vi "Test - Parse Cluster.vi"() -> ()   [LabVIEW 2020, in "JSON Schema Generator.lvlib"]
uses:
  JSON Schema Generator.lvlib
  <vilib>/addons/_JKI Toolkits/Caraya/classes/Test/Test.lvclass
  <vilib>/addons/_JKI Toolkits/Caraya/classes/Assert/Assert.lvclass
  <vilib>/JDP Science/JSONtext/JSONtext.lvlib
  <vilib>/addons/_JKI Toolkits/Caraya/classes/Assert/Assert Equal Value_Variant.vi
  <vilib>/addons/_JKI Toolkits/Caraya/classes/Assert/Assert Not Error.vi
panel:
  out "Typedef Name":string
  out "JSON Object Name":string
  in  "A Cluster":T1
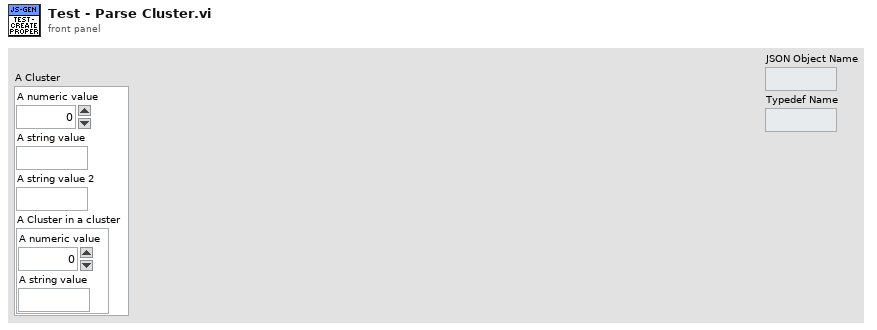
[diagram p1: front panel]
types:
  T1 = cluster{"A numeric value":i32, "A string value":string, "A string value 2":string, "A Cluster in a cluster":cluster{"A numeric value":i32, "A string value":string}}
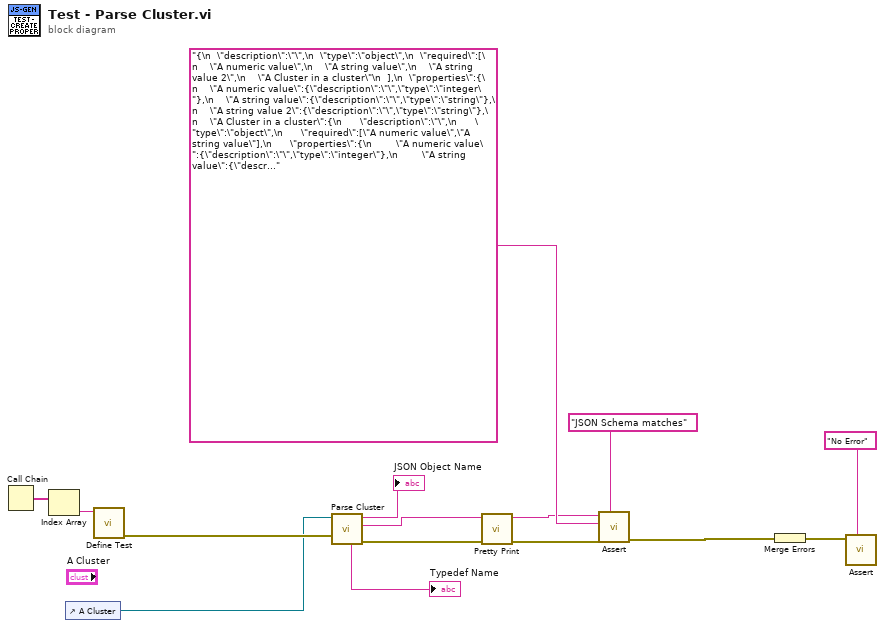
[diagram p0: block diagram]
diagram:
  n1 = Call Chain() -> (call chain=w15:string[])
  n2 = Index Array(array=w15) -> (element=w14:string)  [unwired: 1 in]
  n3 = control-ref of="A Cluster"() -> (w3:refnum<vi>)
  n4 = call <vilib>:"Define Test.vi"("Label (VI Title)"=w14) -> ("error out"=w9:errorcluster)  [unwired: 9 in, 1 out]
  n5 = call "Parse Cluster.vi"("error in"=w9, "Cluster Refnum In"=w3) -> ("error out"=w5:errorcluster, "JSON ObjectSchema out"=w8:string, "JSON Object Name"=→"JSON Object Name":string, "Typedef Name"=→"Typedef Name":string)  [unwired: 5 in, 1 out]
  n6 = call <vilib>:"Pretty Print.vi"("error in (no error)"=w5, "JSON"=w8) -> ("error out"=w4:errorcluster, "<JSON>"=w6:string)  [unwired: 7 in, 1 out]
  n7 = call-poly <vilib>:"Assert.vi"("Label"="JSON Schema matches", "error in (no error)"=w4, "Actual"="{\n  \"description\":\"\",\n  \"type\":\"object\",\n  \"required\":[\n    \"A numeric value\",\n    \"A string value\",\n    \"A string value 2\",\n    \"A Cluster in a cluster\"\n  ],\n  \"properties\":{\n    \"A numeric value\":{\"description\":\"\",\"type\":\"integer\"},\n    \"A string value\":{\"description\":\"\",\"type\":\"string\"},\n    \"A string value 2\":{\"description\":\"\",\"type\":\"string\"},\n    \"A Cluster in a cluster\":{\n      \"description\":\"\",\n      \"type\":\"object\",\n      \"required\":[\"A numeric value\",\"A string value\"],\n      \"properties\":{\n        \"A numeric value\":{\"description\":\"\",\"type\":\"integer\"},\n        \"A string value\":{\"description\":\"\",\"type\":\"string\"}\n      }\n    }\n  }\n}" ("JSON SChema out"), "Expected"=w6) -> ("error out"=w10:errorcluster)  [unwired: 6 in, 1 out]
  n8 = Merge Errors(w10) -> (w11:errorcluster)
  n9 = call-poly <vilib>:"Assert.vi"("Label"="No Error", "Not Error?"=w11) -> ()  [unwired: 8 in, 2 out]
